vi "Chirp Function.vi"(1 "milliseconds to wait":u32, 2 "Amplitude slope":dbl, 3 "Frequency multiplier":dbl, 4 "Resolution":dbl) -> (0 "Chirp Array":dbl[](array[numeric]))   [LabVIEW 2014]
panel:
  out "Chirp Chart":dbl(graph)
  in  "stop":bool
  # "8"
  # "0.01"
  # "0.015"
  # "10"
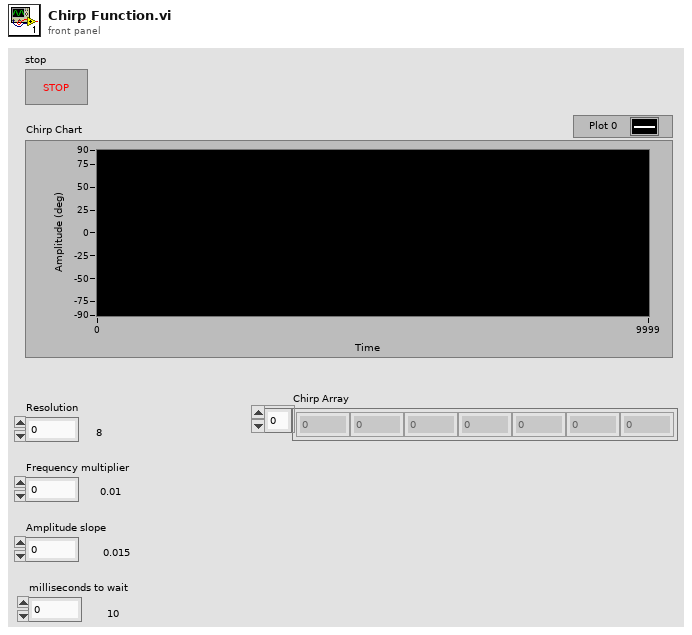
[diagram p1: front panel]
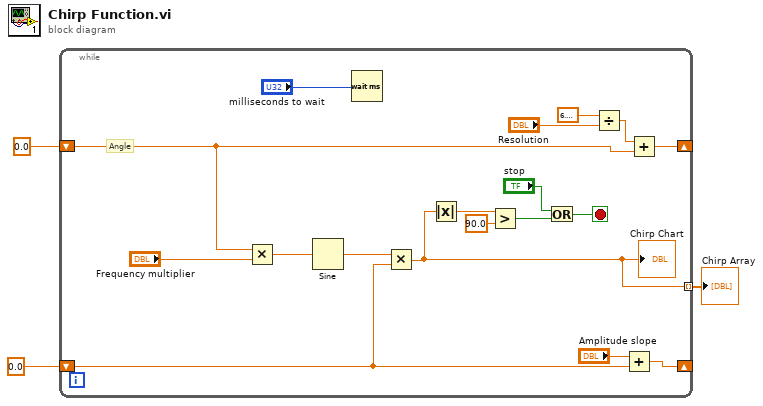
[diagram p0: block diagram]
diagram:
  n1 = while {
    shift-right: [w21] -> _
    shift-left: 0.0 -> [w16]
    shift-right: [w14] -> _
    shift-left: 0.0 -> [w11]
    tunnel: [w5] -> w1 mode=indexing
    stop <- w6 stop-if-true
    # "Angle"
    n2 = Multiply(x=w16, y="Frequency multiplier") -> (x*y=w17:dbl)
    n3 = Sine(x=w17) -> (sin(x)=w12:dbl)
    n4 = Wait (ms)(milliseconds to wait="milliseconds to wait") -> ()  [unwired: 1 out]
    n5 = Multiply(x=w12, y=w11) -> (x*y=w5:dbl)
    "Chirp Chart" <- w5
    n6 = Absolute Value(x=w5) -> (abs(x)=w10:dbl)
    n7 = Greater?(x=w10, y=90.0) -> (0:w8:bool)
    n8 = Or(x="stop", y=w8) -> (x .or. y?=w6:bool)
    n9 = Divide(x=6.283185307179586, y="Resolution") -> (x/y=w20:dbl)
    n10 = Add(x="Amplitude slope", y=w11) -> (x+y=w14:dbl)
    n11 = Add(x=w20, y=w16) -> (x+y=w21:dbl)
  }
  "Chirp Array" <- w1
